vi "_RT_CtrlLoop_SigTrnsfr_Conv_IP.vi"(1 "EndPoint":string) -> (0 "IP/Endpoint":string)   [LabVIEW 2018]
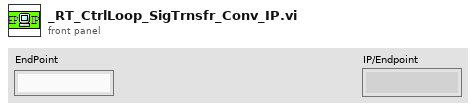
[diagram p1: front panel]
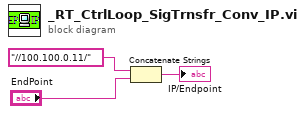
[diagram p0: block diagram]
diagram:
  n1 = Concatenate Strings("//100.100.0.11/", "EndPoint") -> (→"IP/Endpoint":string)
